vi "Get Entry.vi"(8 "error in (no error)":errorcluster, 10 "Key":string caption="Name", 11 "Registry in":refnum<class "Registry.lvclass">) -> (0 "error out":errorcluster, 1 "Value":variant, 2 "Key Out":string caption="Name Out", 4 "Found?":bool)   [LabVIEW 2020, in "BCI-1553 API.lvlib" / "Registry.lvlib" / "Registry.lvclass"]
doc: "Retrieves a Key/Value pair from the Registry."
uses:
  Registry.lvclass
  Registry.lvclass/Registry.ctl
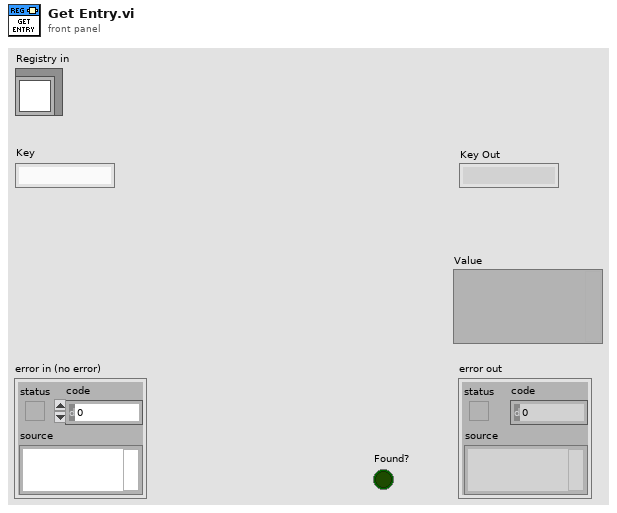
[diagram p1: front panel]
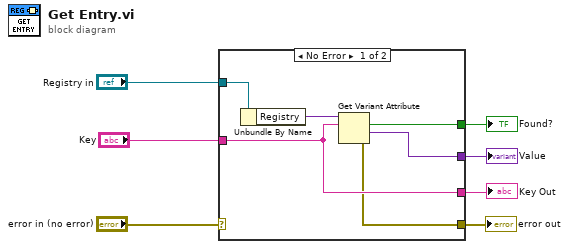
[diagram p0: block diagram]
diagram:
  n1 = case shown="No Error" "error in (no error)" {
    selector: "error in (no error)" -> [_ w14]
    tunnel: [w9 w14] -> w6
    tunnel: "Registry in" -> [w13 _]
    tunnel: "Key" -> [w10 _]
    tunnel: [w12 _] -> w3
    tunnel: [w11 _] -> w2
    tunnel: [w10 _] -> w1
    frame No Error {
      n2 = Unbundle By Name(w13) -> ("Registry"=w8:variant)
      n3 = Get Variant Attribute(Variant=w8, name=w10) -> (found=w12:bool, value=w11:variant, error out=w9:errorcluster)  [unwired: 2 in, 1 out]
    }
    frame Error {
    }
  }
  "error out" <- w6
  "Found?" <- w3
  "Value" <- w2
  "Key Out" <- w1
